vi "close all.vi"(8 "error in (no error)":errorcluster, 11 "USRP_1_x_200MHz in":refnum<class "USRP_1_x_200MHz.lvclass">) -> (0 "error out":errorcluster, 3 "USRP_1_x_200MHz out":refnum<class "USRP_1_x_200MHz.lvclass">)   [LabVIEW 2021, in "USRP_1_x_200MHz.lvclass"]
uses:
  USRP_1_x_200MHz.lvclass
  USRP_1_x_200MHz.lvclass/USRP_1_x_200MHz.ctl
  <vilib>/FPGAPlugInAG/Dynamic/niLvFpga_Close_Dynamic.vi
  <vilib>/rvi/interface/nirviCloseFPGA/nirviCloseFPGA.xnode
  <instrlib>/niUsrpRio/Config/v1/Host/niUsrpRio Config v1 Host.lvlib
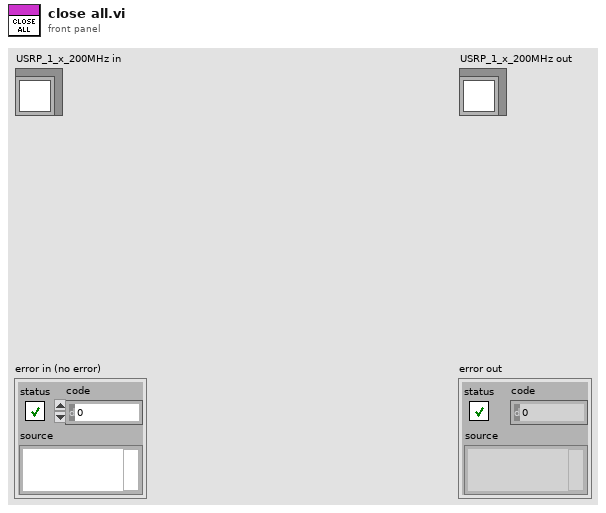
[diagram p1: front panel]
types:
  T1 = typedef "niUsrpRio Config v1 Host.lvlib/niUsrpRio Session.ctl" = cluster{"FPGA Interface":refnum<k20>, "RIO Interface Number":u32, "Data Clock Rate":u32, "FPGA Data Clock Rate":u32, "Global Settings Register Bus":T2, "Radio 0 Settings Register Bus":T2, "Radio 1 Settings Register Bus":T2, "Radio Settings Bus Semaphore":T3, "DB Queues":T4[], "Characterization Data Valid?":bool, "EEPROM Header":T5, "Device Data Header":T6, "EEPROM Characterization Header":T7, "Characterization Data":T8[], "FPGA Current Version":u32, "FPGA Oldest Compatible Version":u32, "Fixed Logic Current Version":u32, "Fixed Logic Oldest Compatible Version":u32, "FPGA Radio Settings Bus Current Version":u32, "FPGA Radio Settings Bus Oldest Compatible Version":u32, "FPGA Board Config Current Version":u32, "FPGA Board Config Oldest Compatible Version":u32, "Daughterboard Clock Rate":u32, "daughterboard configuration session handles":u64[]}
  T2 = typedef "niInstr Register Bus v0 Host.lvlib/Register Bus Session.ctl" = refnum<queue>
  T3 = typedef "Semaphore RefNum" = refnum<k1>
  T4 = typedef "niUsrpRio Config v1 Host.lvlib/DB Queue Reference.ctl" = refnum<queue>
  T5 = typedef "niUsrpRio Config v1 Host.lvlib/EEPROM Header.ctl" = cluster{"Checksum":u32, "Product Code":u16, "Hardware Current Version":u16, "Hardware Oldest Compatible Version":u16, "EEPROM Map Current Version":u16, "EEPROM Map Oldest Compatible Version":u16, "User Password":string, "Pointer to Factory Header":u32, "Pointer to User Header":u32, "Recommended Interval":u16, "Number of Reserved Bytes":i32, "Number of Daughterboards":u8, "Daughterboard IDs":u16[], "Daughterboard Serial Numbers":string[]}
  T6 = typedef "niUsrpRio Config v1 Host.lvlib/EEPROM Device Data Header.ctl" = cluster{"Checksum":u32, "Number of Channels":u8, "Number of Gain Settings":u16[], "Pointer to Characterization Data":u32[], "Number of Reserved Bytes":i32, "Number of Frequencies":u16[]}
  T7 = typedef "niUsrpRio Config v1 Host.lvlib/EEPROM Characterization Header.ctl" = cluster{"Checksum":u32, "Date":timestamp, "Temperature":sgl, "Misc. Info":string, "Pointer to Device Data Header":u32, "Number of Reserved Bytes":i32}
  T8 = typedef "niUsrpRio Config v1 Host.lvlib/Characterization Data.ctl" = cluster{"Gains[dB]":dbl[], "Frequencies [Hz]":dbl[], "IQ Imbalance Table":T9[], "Measured Gains[dB]":dbl[][]}
  T9 = typedef "niUsrpRio Config v1 Host.lvlib/IQ Imbalance.ctl" = cluster{"Gain Imbalance [linear]":dbl, "Phase Imbalance [radians]":dbl, "Offset":cdb}
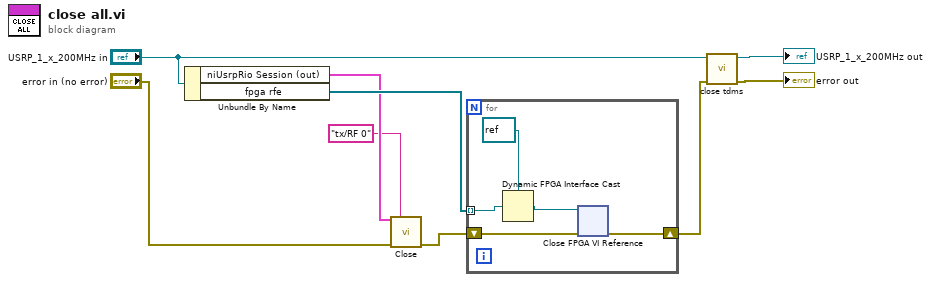
[diagram p0: block diagram]
diagram:
  n1 = Unbundle By Name("USRP_1_x_200MHz in") -> ("niUsrpRio Session (out)"=w8:T1, "fpga rfe"=w9:refnum<k20>[])
  n2 = call <instrlib>:"Close.vi"("niUsrpRio Session"=w8, "scope"="tx/RF 0", "error in"="error in (no error)") -> ("error out"=w6:errorcluster)  [unwired: 11 in, 1 out]
  n3 = for {
    shift-right: [w13] -> w3
    shift-left: w6 -> [w14]
    tunnel: w9 -> [w12] mode=indexing
    n4 = Dynamic FPGA Interface Cast(Session In=refnum<k20> refnum ("FPGA VI Reference Out"), Type=w12) -> (Session Out=w10:refnum<k20>)
    n5 = xnode "Close FPGA VI Reference"("FPGA VI Reference In"=w10, "error in"=w14) -> ("error out"=w13:errorcluster)
  }
  n6 = call-dynamic "close tdms.vi"("error in (no error)"=w3, "device_type in"="USRP_1_x_200MHz in") -> ("error out"=→"error out":errorcluster, "device_type out"=→"USRP_1_x_200MHz out":refnum<class "USRP_1_x_200MHz.lvclass">)  [unwired: 8 in]
